vi "Format InstanceStateType_LVXML_Loop.vi"(8 "error in (no error)":errorcluster, 11 "Siblings in":T2(array[cluster])) -> (0 "error out":errorcluster, 3 "Array":T3[](array[typedef]))   [LabVIEW 2014, in "AWS_EC2.lvlib" / "AWS_EC2.lvclass"]
uses:
  AWS_EC2.lvclass
  EC2 Datatypes/InstanceStatusDetailsSetType.ctl
  lv-xml-parser/r0/trunk/VI Source/EventType.ctl
  lv-xml-parser/r0/trunk/VI Source/LV XML Parser.lvlib
  AWS_EC2.lvlib
  AWS Core Lib/VI Source/AWS_Core.lvlib
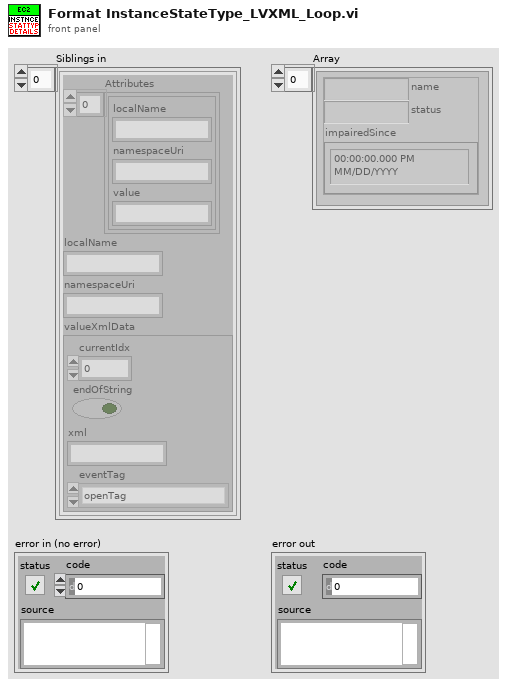
[diagram p1: front panel]
types:
  T1 = typedef "LV XML Parser.lvlib/EventType.ctl" = enum16{"openTag", "endOpenTag", "closeTag", "comment", "endComment", "endOfFile", "attribute", "startXml"}
  T2 = cluster{"Attributes":cluster{"localName":string, "namespaceUri":string, "value":string}[], "localName":string, "namespaceUri":string, "valueXmlData":cluster{"currentIdx":i32, "endOfString":bool, "xml":string, "eventTag":T1}}[]
  T3 = typedef "AWS_EC2.lvlib/InstanceStatusDetailsSetType.ctl" = cluster{"name":string, "status":string, "impairedSince":timestamp}
  T4 = cluster{"Attributes":cluster{"localName":string, "namespaceUri":string, "value":string}[], "localName":string, "namespaceUri":string, "valueXmlData":cluster{"currentIdx":i32, "endOfString":bool, "xml":string, "eventTag":T1}}
  T5 = cluster{"currentIdx":i32, "endOfString":bool, "xml":string, "eventTag":T1}
  T6 = cluster{"namespaceUri":string, "localName":string}
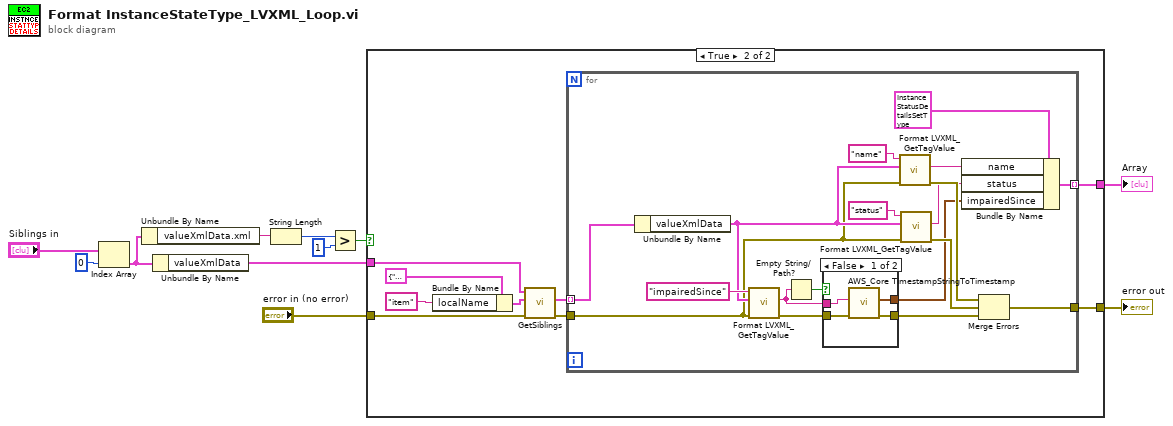
[diagram p0: block diagram]
diagram:
  n1 = Index Array(array="Siblings in", index=0) -> (element=w1:T4)
  n2 = Unbundle By Name(w1) -> ("valueXmlData.xml"=w2:string)
  n3 = Unbundle By Name(w1) -> ("valueXmlData"=w8:T5)
  n4 = String Length(string=w2) -> (length=w4:i32)
  n5 = Greater?(x=w4, y=1) -> (0:w9:bool)
  n6 = case shown="True" w9 {
    tunnel: "error in (no error)" -> [w12 w18]
    tunnel: w8 -> [_ w17]
    tunnel: [w12 w13] -> w11
    tunnel: [_ w14] -> w10
    frame False {
    }
    frame True {
      n7 = Bundle By Name(cluster=T6 {"namespaceUri"="", "localName"=""} ("limitToTag"), "localName"="item" ("Tag name")) -> (w20:T6)
      n8 = call "GetSiblings.vi"("error in (no error)"=w18, "limitToTag"=w20, "xmlData"=w17) -> ("error out"=w16:errorcluster, "Siblings"=w15:T2)  [unwired: 7 in]
      n9 = for {
        tunnel: w16 -> [w26]
        tunnel: w15 -> [w37] mode=indexing
        tunnel: [w38] -> w14 mode=indexing
        tunnel: [w34] -> w13
        n10 = Unbundle By Name(w37) -> ("valueXmlData"=w29:T5)
        n11 = call "Format LVXML_GetTagValue.vi"("error in (no error)"=w26, "xmlDataIn"=w29, "Tag name"="impairedSince") -> ("error out"=w27:errorcluster, "Value"=w22:string)  [unwired: 6 in, 1 out]
        n12 = Empty String/Path?(string/path=w22) -> (empty?=w23:bool)
        n13 = case shown="False" w23 {
          tunnel: [w43 _] -> w28
          tunnel: w27 -> [w42 w44]
          tunnel: [w41 w44] -> w25
          tunnel: w22 -> [w40 _]
          frame False {
            n14 = call "AWS_Core TimestampStringToTimestamp.vi"("error in"=w42, "AWS Timestamp String"=w40) -> ("error out"=w41:errorcluster, "Time Stamp Control"=w43:timestamp)  [unwired: 8 in]
          }
          frame True {
          }
        }
        n15 = call "Format LVXML_GetTagValue.vi"("error in (no error)"=w26, "xmlDataIn"=w29, "Tag name"="name") -> ("error out"=w32:errorcluster, "Value"=w33:string)  [unwired: 6 in, 1 out]
        n16 = call "Format LVXML_GetTagValue.vi"("error in (no error)"=w26, "xmlDataIn"=w29, "Tag name"="status") -> ("error out"=w31:errorcluster, "Value"=w24:string)  [unwired: 6 in, 1 out]
        n17 = Bundle By Name(cluster=T3 {"name"="", "status"="", "impairedSince"=timestamp(0 s since 1904-01-01)} ("InstanceStatusDetailsSetType"), "name"=w33, "status"=w24, "impairedSince"=w28) -> (w38:T3)
        n18 = Merge Errors(w32, w31, w25) -> (w34:errorcluster)
      }
    }
  }
  "error out" <- w11
  "Array" <- w10
